vi "niFpgaGenerateCodeResults_Paths.vi"() -> ()   [LabVIEW 2020]
panel:
  in  "signatureTags":T1={"signatureRoot"="signatures", "fpgaSignature"="fpgaSignature", "guidSignature"="guidSignature", "nameSignature"="namesSignature"}
  in  "simulationTags":T2={"simulationRoot"="simulation", "topLvlSimulationModel"="topLvlModName", "genSimCode"="genSimulationCode", "exportedSignals"={"exportClip"="exportClip", "exportNipi"="exportNipi", "exportEio"="exportEio", "exportTopLvl"="exportTopLvl"}}
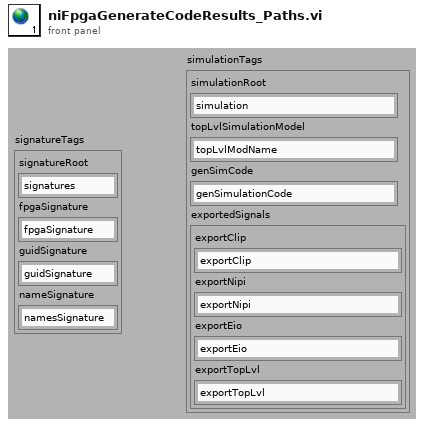
[diagram p1: front panel]
types:
  T1 = cluster{"signatureRoot":string, "fpgaSignature":string, "guidSignature":string, "nameSignature":string}
  T2 = cluster{"simulationRoot":string, "topLvlSimulationModel":string, "genSimCode":string, "exportedSignals":cluster{"exportClip":string, "exportNipi":string, "exportEio":string, "exportTopLvl":string}}
diagram:
